vi "Get Ctl Refnum By Label.vi"(8 "error in":errorcluster, 10 "Label":string, 11 "Main Data Buffer In":T1) -> (0 "error out":errorcluster, 2 "Ctl Refnum":refnum<vi>, 3 "Main Data Buffer Out":T1)   [LabVIEW 2020, in "SECS Bridge.lvlib"]
uses:
  SECS Bridge.lvlib
  Main Data Buffer.ctl
  SECS Communication/HSMS Class/HSMS Class.lvclass
  SECS Communication/SECS Data Class/SECS Data Class.lvclass
  SECS Scenarios/Scenarios Class/Scenarios Class.lvclass
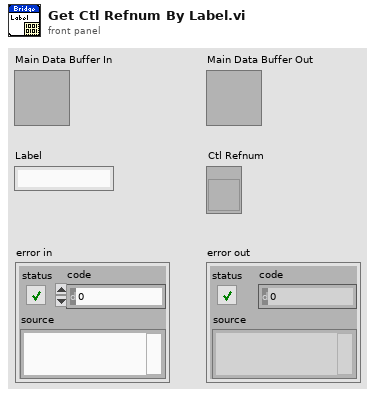
[diagram p1: front panel]
types:
  T1 = typedef "SECS Bridge.lvlib/Main Data Buffer.ctl" = cluster{"HSMS Class":refnum<class "HSMS Class.lvclass">, "SECS Data Class":refnum<class "SECS Data Class.lvclass">, "Scenarios Class":refnum<class "Scenarios Class.lvclass">, "VI Refnum":refnum<vi>, "Ctl Refnum Map":map{string, refnum<vi>}, "Timeout":i32, "Notifier Data":string[], "Event Refnum":refnum<event-registration>}
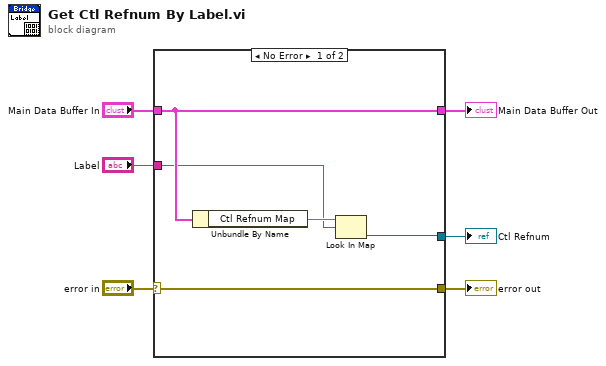
[diagram p0: block diagram]
diagram:
  n1 = case shown="No Error" "error in" {
    selector: "error in" -> [w11 w12]
    tunnel: [w11 w12] -> w5
    tunnel: "Main Data Buffer In" -> [w10 w13]
    tunnel: [w10 w13] -> w3
    tunnel: "Label" -> [w8 _]
    tunnel: [w7 _] -> w1
    frame No Error {
      n2 = Unbundle By Name(w10) -> ("Ctl Refnum Map"=w9:map{string, refnum<vi>})
      n3 = Look In Map(map=w9, key=w8) -> (value=w7:refnum<vi>)  [unwired: 1 in, 1 out]
    }
    frame Error {
    }
  }
  "error out" <- w5
  "Main Data Buffer Out" <- w3
  "Ctl Refnum" <- w1
